vi "DeMux16.vi"(1 "X":bool, 2 "S":bool[](array[boolean])) -> (0 "A":bool[](array[boolean]))   [LabVIEW 2012]
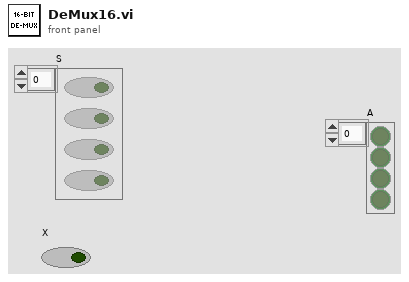
[diagram p1: front panel]
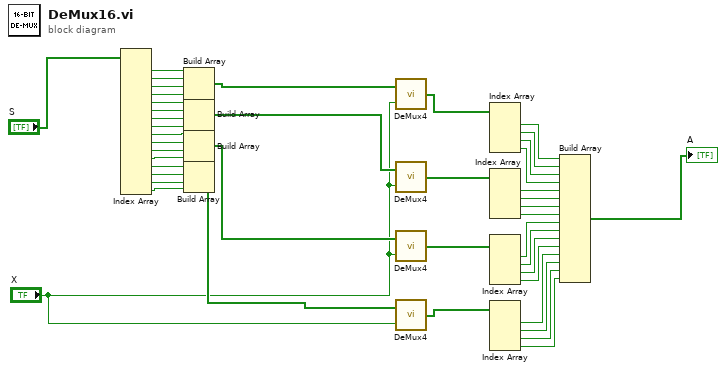
[diagram p0: block diagram]
diagram:
  n1 = Index Array(array="S") -> (element #1=w43:bool, element #2=w42:bool, element #3=w41:bool, element #4=w40:bool, element #5=w39:bool, element #6=w38:bool, element #7=w37:bool, element #8=w36:bool, element #9=w35:bool, element #10=w34:bool, element #11=w33:bool, element #12=w32:bool, element #13=w31:bool, element #14=w30:bool, element #15=w29:bool, element #16=w28:bool)  [unwired: 16 in]
  n2 = Build Array(w43, w42, w41, w40) -> (w27:bool[])
  n3 = Build Array(w39, w38, w37, w36) -> (w26:bool[])
  n4 = Build Array(w35, w34, w33, w32) -> (w25:bool[])
  n5 = Build Array(w31, w30, w29, w28) -> (w24:bool[])
  n6 = call "DeMux4.vi"("X"="X", "S"=w27) -> ("A"=w7:bool[])
  n7 = call "DeMux4.vi"("X"="X", "S"=w26) -> ("A"=w6:bool[])
  n8 = call "DeMux4.vi"("X"="X", "S"=w25) -> ("A"=w5:bool[])
  n9 = call "DeMux4.vi"("X"="X", "S"=w24) -> ("A"=w4:bool[])
  n10 = Index Array(array=w7) -> (element #1=w23:bool, element #2=w22:bool, element #3=w21:bool, element #4=w20:bool)  [unwired: 4 in]
  n11 = Index Array(array=w6) -> (element #1=w19:bool, element #2=w18:bool, element #3=w17:bool, element #4=w16:bool)  [unwired: 4 in]
  n12 = Index Array(array=w5) -> (element #1=w15:bool, element #2=w14:bool, element #3=w13:bool, element #4=w12:bool)  [unwired: 4 in]
  n13 = Index Array(array=w4) -> (element #1=w11:bool, element #2=w10:bool, element #3=w9:bool, element #4=w8:bool)  [unwired: 4 in]
  n14 = Build Array(w23, w22, w21, w20, w19, w18, w17, w16, w15, w14, w13, w12, w11, w10, w9, w8) -> (→"A":bool[])
